vi "F510.vi"   [LabVIEW 2015]
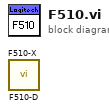
[diagram p0: block diagram]
diagram:
  n1 = call "F510-D.vi"() -> ()  [unwired: 7 in, 5 out]
  n2 = call "F510-X.vi"() -> ()  [unwired: 5 in, 7 out]
